vi "Load Signal Bank (by channel num).vi"(4 "error in (no error)":errorcluster, 5 "Input array":dbl[][](array[numeric])=array10000x1[10000 elements] format="%.2f", 6 "Active AO Array":u16[](array[numeric]), 7 "timeout (ms)":i32=5000) -> (0 "error out":errorcluster={"status"=FALSE, "code"=0, "source"="."})   [LabVIEW 2015]
uses:
  DAQ Engine VIs/PXI Globals.vi
panel:
  out "Waveform Graph":dbl[][](graph)
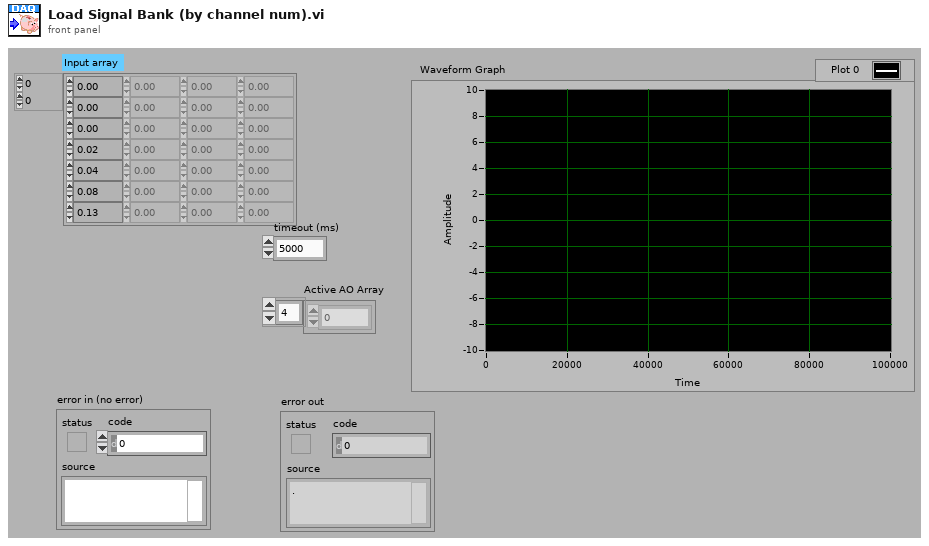
[diagram p1: front panel]
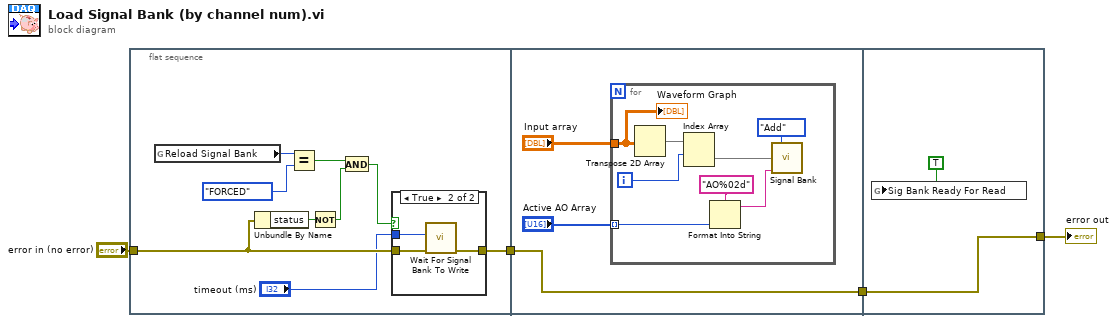
[diagram p0: block diagram]
diagram:
  n1 = flat-sequence {
    tunnel: "error in (no error)" -> [w6]
    tunnel: [w13] -> w3
    tunnel: w3 -> [w20]
    tunnel: [w20] -> w2
    tunnel: [w29] -> w1
    tunnel: w2 -> [w29]
    frame #0 {
      n2 = global read "PXI Globals.vi" "Reload Signal Bank"() -> (w8:enum32{"OFF", "ENABLED", "FORCED"})
      n3 = Unbundle By Name(w6) -> ("status"=w10:bool)
      n4 = Equal?(x=w8, y=enum16{"OFF", "ENABLED", "FORCED"}."FORCED") -> (x = y?=w12:bool)
      n5 = Not(x=w10) -> (.not. x?=w11:bool)
      n6 = And(x=w12, y=w11) -> (x .and. y?=w7:bool)
      n7 = case shown="True" w7 {
        tunnel: w6 -> [w14 w17]
        tunnel: [w14 w16] -> w13
        tunnel: "timeout (ms)" -> [_ w15]
        frame False {
        }
        frame True {
          n8 = call "Wait For Signal Bank To Write.vi"("error in (no error)"=w17, "timeout (ms)"=w15) -> ("error out"=w16:errorcluster)  [unwired: 8 in, 1 out]
        }
      }
    }
    frame #1 {
      n9 = for {
        tunnel: "Active AO Array" -> [w27] mode=indexing
        tunnel: "Input array" -> [w21]
        i -> [w25]
        n10 = Transpose 2D Array(2D array=w21) -> (transposed array=w24:dbl[][])
        n11 = Index Array(array=w24, index (row)=w25) -> (element=w23:dbl[])  [unwired: 1 in]
        n12 = Format Into String(format string="AO%02d", w27) -> (resulting string=w26:string)  [unwired: 2 in, 1 out]
        n13 = call "Signal Bank.vi"("Action"=enum16{"Add", "Replace ID", "Read ID", "Clear"}."Add", "1D Data In"=w23, "ID"=w26) -> ()  [unwired: 11 in, 2 out]
        "Waveform Graph" <- w21
      }
    }
    frame #2 {
      n14 = global write "PXI Globals.vi" "Sig Bank Ready For Read"(TRUE) -> ()
    }
  }
  "error out" <- w1
